vi "microStepLoop_backup_with_crio_code.vi"(6 "Corrected_increment":i32, 9 "Trigger":bool, 10 "reset_ustep_x":bool, 11 "steps_in_a_ramp_x in":i32) -> (0 "Condition for microstep loop":bool, 1 "currentUstep":i32, 2 "nextUstep":i32, 3 "botRamp":bool, 4 "TopRamp":bool, 5 "maxPulse":bool)   [LabVIEW 2016]
panel:
  in  "CorrectedIncrement":i32
  out "bot_ramp_x":bool
  out "max_pulse_x":bool
  in  "resetUstep":bool
  out "next_ustep_x":i32
  out "curent_ustep_x":i32
  out "top_ramp_x":bool
  in  "steps_in_a_ramp_x":i32
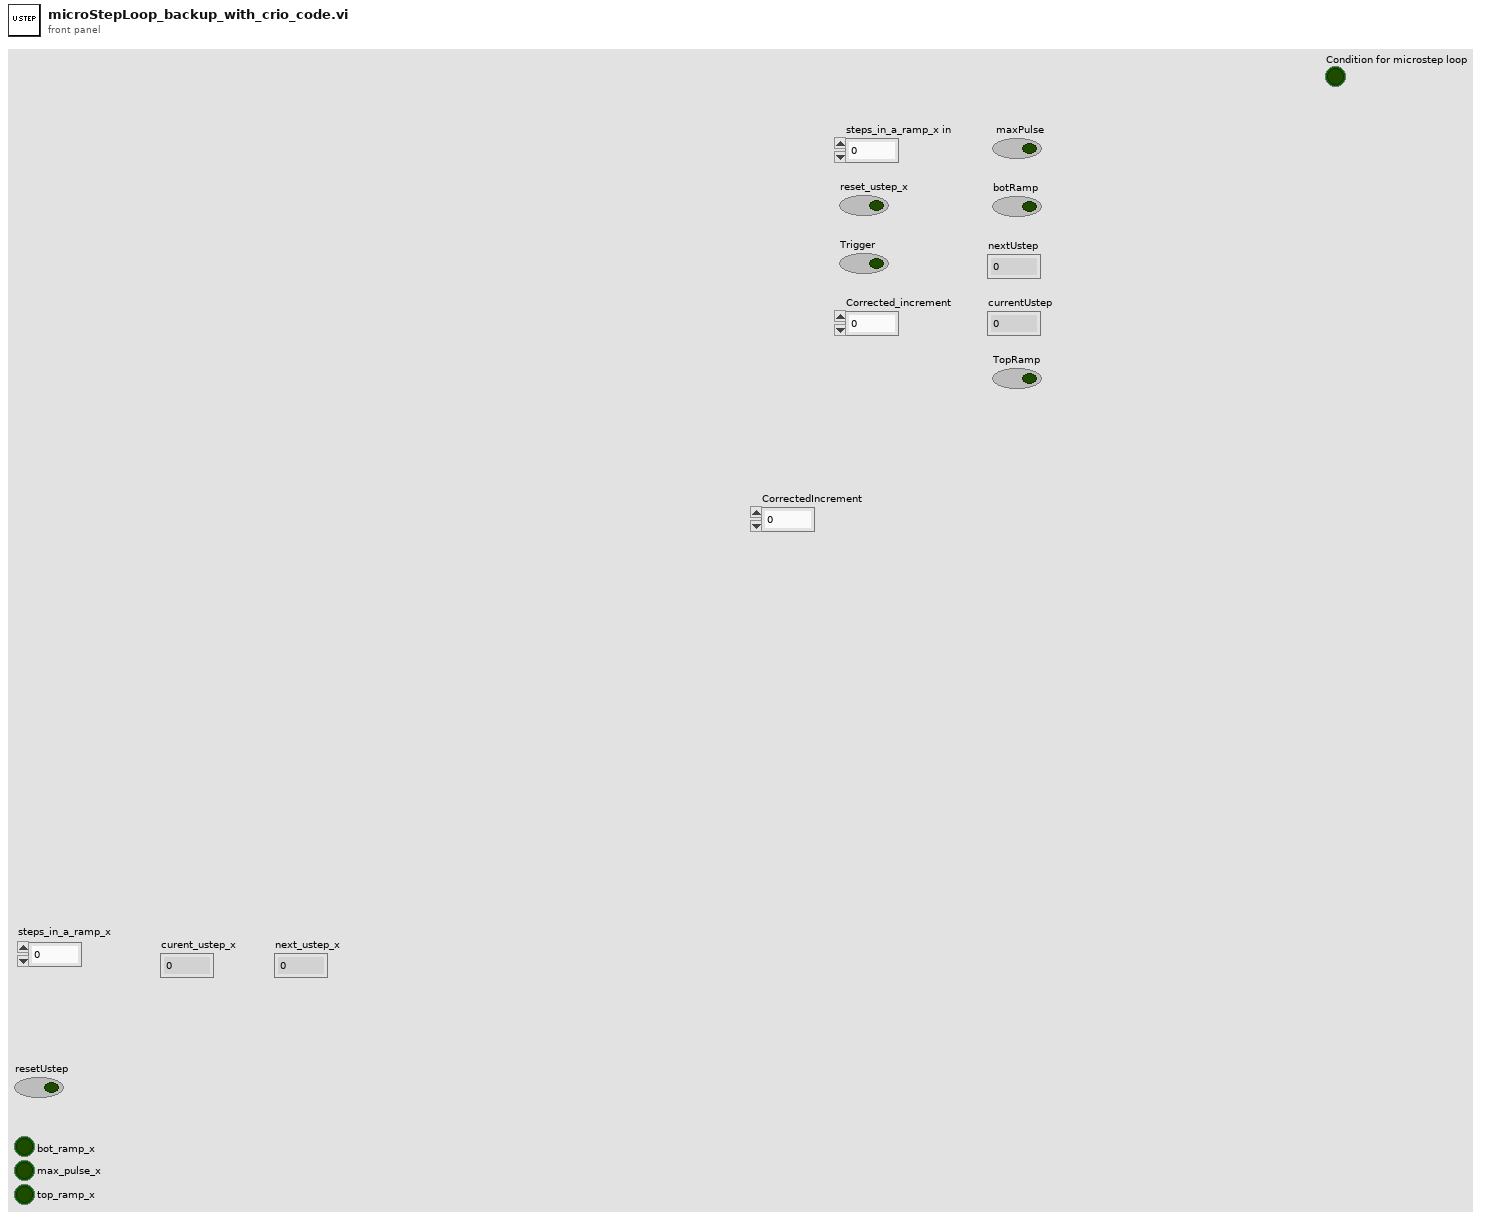
[diagram p1: front panel]
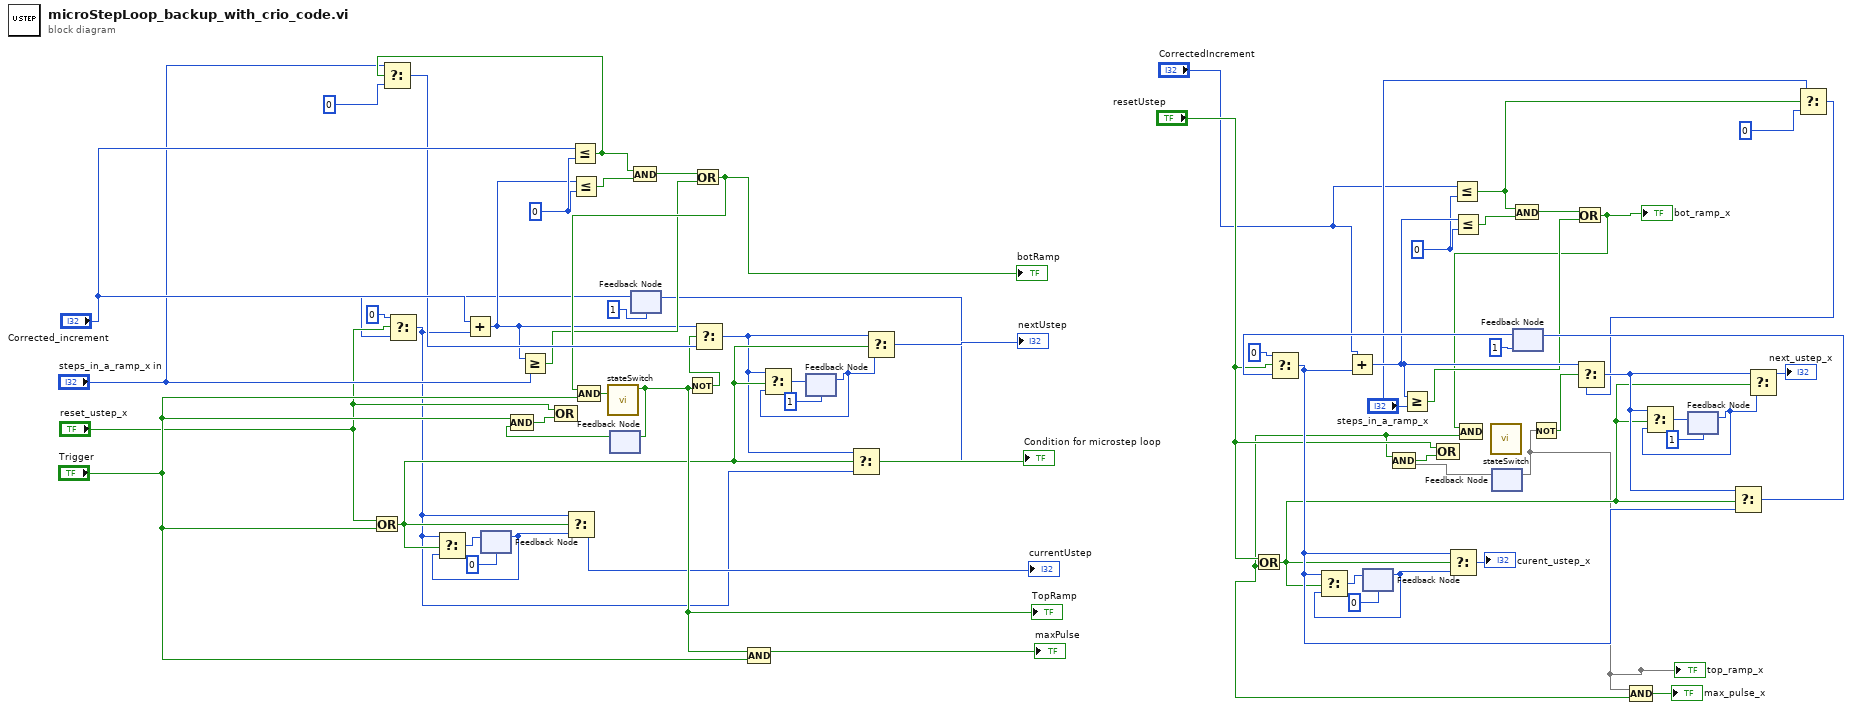
[diagram p0: block diagram]
diagram:
  w12 = 0
  w56 = 0
  n1 = Or(x="reset_ustep_x", y="Trigger") -> (x .or. y?=w49:bool)
  "Condition for microstep loop" <- w49
  n2 = feedback #1(0 ("t")) -> (w42:i32)
  n3 = Less Or Equal?(x="Corrected_increment", y=w56) -> (x <= y?=w64:bool)
  n4 = Select(t="steps_in_a_ramp_x in", s=w64, f=0) -> (s? t:f=w63:i32)
  n5 = feedback #2() -> (w51:bool)  [unwired: 1 in]
  n6 = Compound Arithmetic op=AND("Trigger", w51) -> (w50:bool)
  n7 = Compound Arithmetic op=OR("reset_ustep_x", w50) -> ()  [unwired: 1 out]
  n8 = feedback #3(1) -> (w36:i32)
  n9 = Select(t=0, s="reset_ustep_x", f=w36) -> (s? t:f=w41:i32)
  n10 = Select(t=w41, s=w49, f=w42) -> (s? t:f=w40:i32)
  n11 = Add(x="Corrected_increment", y=w41) -> (x+y=w55:i32)
  n12 = feedback-in #1(w40) -> ()
  n13 = Greater Or Equal?(x=w55, y="steps_in_a_ramp_x in") -> (x >= y?=w58:bool)
  n14 = Select(t=w41, s=w49, f=w42) -> (s? t:f=→"currentUstep":i32)
  n15 = Less Or Equal?(x=w55, y=w56) -> (x <= y?=w57:bool)
  n16 = And(x=w64, y=w57) -> (x .and. y?=w59:bool)
  n17 = Or(x=w59, y=w58) -> (x .or. y?=w60:bool)
  "botRamp" <- w60
  n18 = Compound Arithmetic op=AND(w60, "Trigger") -> (w1:bool)
  n19 = call "stateSwitch.vi"("enable"=w1) -> ("state"=w65:bool)  [unwired: 10 in]
  "TopRamp" <- w65
  n20 = feedback-in #2(w65) -> ()
  n21 = Not(x=w65) -> (.not. x?=w52:bool)
  n22 = Select(t=w55, s=w52, f=w63) -> (s? t:f=w43:i32)
  n23 = Compound Arithmetic op=AND(w65, "Trigger") -> (→"maxPulse":bool)
  n24 = feedback #4(1) -> (w45:i32)
  n25 = Select(t=w43, s=w49, f=w45) -> (s? t:f=w44:i32)
  n26 = feedback-in #4(w44) -> ()
  n27 = Select(t=w43, s=w49, f=w41) -> (s? t:f=w37:i32)
  n28 = feedback-in #3(w37) -> ()
  n29 = Select(t=w43, s=w49, f=w45) -> (s? t:f=→"nextUstep":i32)
  n30 = feedback #5(0 ("t")) -> (w27:i32)
  n31 = Less Or Equal?(x="CorrectedIncrement", y=w12) -> (x <= y?=w4:bool)
  n32 = call "stateSwitch.vi"() -> ()  [unwired: 11 in, 1 out]
  n33 = feedback #6() -> (w18)  [unwired: 1 in]
  n34 = feedback-in #6() -> (w15)
  "top_ramp_x" <- w15
  n35 = feedback #7(1) -> (w33:i32)
  n36 = Select(t=0, s="resetUstep", f=w33) -> (s? t:f=w28:i32)
  n37 = Add(x="CorrectedIncrement", y=w28) -> (x+y=w13:i32)
  n38 = Greater Or Equal?(x=w13, y="steps_in_a_ramp_x") -> (x >= y?=w10:bool)
  n39 = Less Or Equal?(x=w13, y=w12) -> (x <= y?=w11:bool)
  n40 = And(x=w4, y=w11) -> (x .and. y?=w9:bool)
  n41 = Not(x=w15) -> (.not. x?=w17:bool)
  n42 = Or(x=w9, y=w10) -> (x .or. y?=w8:bool)
  "bot_ramp_x" <- w8
  n43 = Compound Arithmetic op=AND(w8) -> (w3:bool)  [unwired: 1 out]
  n44 = Or(x="resetUstep", y=w3) -> (x .or. y?=w20:bool)
  n45 = Select(t=w28, s=w20, f=w27) -> (s? t:f=w29:i32)
  n46 = feedback-in #5(w29) -> ()
  n47 = Compound Arithmetic op=AND(w3, w18) -> (w19:bool)
  n48 = Compound Arithmetic op=OR("resetUstep", w19) -> ()  [unwired: 1 out]
  n49 = Select(t=w28, s=w20, f=w27) -> (s? t:f=→"curent_ustep_x":i32)
  n50 = Compound Arithmetic op=AND(w15, w3) -> (→"max_pulse_x":bool)
  n51 = feedback #8(1) -> (w24:i32)
  n52 = Select(t="steps_in_a_ramp_x", s=w4, f=0) -> (s? t:f=w5:i32)
  n53 = Select(t=w13, s=w17, f=w5) -> (s? t:f=w26:i32)
  n54 = Select(t=w26, s=w20, f=w24) -> (s? t:f=w25:i32)
  n55 = feedback-in #8(w25) -> ()
  n56 = Select(t=w26, s=w20, f=w28) -> (s? t:f=w32:i32)
  n57 = feedback-in #7(w32) -> ()
  n58 = Select(t=w26, s=w20, f=w24) -> (s? t:f=→"next_ustep_x":i32)
